vi "Gaussian White Noise (obs 90).vi"(2 "seed":i32=-1, 3 "standard deviation":dbl=1.0000000000000002 format="%0.2f", 4 "samples":i32=128) -> (0 "error":i32, 1 "Gaussian noise pattern":dbl[](array[numeric]))   [LabVIEW 2010, in "NI_AALBase.lvlib"]
doc: "The Gaussian White Noise VI was rewritten in LabVIEW 2009. Replace this VI with a Gaussian White Noise VI from the <B>Functions</B> palette to use the new functionality.\n\nGenerates a Gaussian-distributed, pseudorandom pattern whose statistical profile is (micro,sigma) = (0,s), where s is <B>standard deviation</B>.\n\nThe Gaussian White Noise VI generates the Gaussian-distributed pseudorandom sequence using a modified version of the Box-Muller method to transform uniformly distributed random numbers into Gaussian-distributed random numbers. LabVIEW uses a triple-seeded very-long-cycle linear congruential generation (LCG) algorithm to generate the uniform pseudorandom numbers."
uses:
  NI_AALBase.lvlib
  lvanlys.dll
panel:
  # "Gaussian White Noise"
  # "This VI is obsolete !!!\nYou should replace this VI in your diagram with the Gaussian White Noise VI."
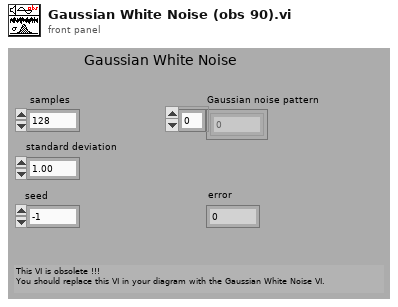
[diagram p1: front panel]
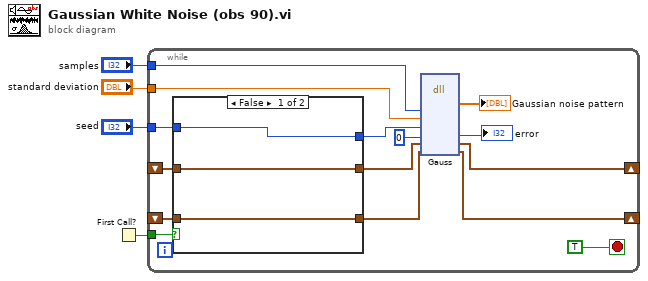
[diagram p0: block diagram]
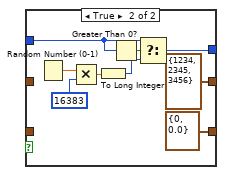
[diagram p2: hidden frame]
diagram:
  n1 = First Call?() -> (First Call?: T/F=w4:bool)
  n2 = while {
    shift-right: [w8] -> _
    shift-left: _ -> [w11]
    tunnel: w4 -> [w5]
    shift-right: [w6] -> _
    shift-left: _ -> [w10]
    tunnel: "seed" -> [w13]
    tunnel: "standard deviation" -> [w15]
    tunnel: "samples" -> [w14]
    stop <- TRUE stop-if-true
    n3 = case shown="False" w5 {
      tunnel: [w21 cluster{"xSeed":i32, "ySeed":i32, "zSeed":i32} {"xSeed"=1234, "ySeed"=2345, "zSeed"=3456} ("RNGState")] -> w9
      tunnel: [w22 w29] -> w12
      tunnel: w13 -> [w22 w30]
      tunnel: [w20 cluster{i32, dbl} {0, 0.0}] -> w7
      tunnel: w11 -> [w21 _]
      tunnel: w10 -> [w20 _]
      frame False {
      }
      frame True {
        n4 = Random Number (0-1)() -> (number: 0 to 1=w27:dbl)
        n5 = Multiply(x=w27, y=16383 ("x")) -> (x*y=w28:dbl)
        n6 = To Long Integer(number=w28) -> (32bit integer=w26:i32)
        n7 = Greater Than 0?(x=w30) -> (x > 0?=w31:bool)
        n8 = Select(t=w30, s=w31, f=w26) -> (s? t:f=w29:i32)
      }
    }
    n9 = dll-call lib="C:/Program Files/National Instruments/LabVIEW 2010/resource/lvanlys.*" fn="Gauss"("size"=w14, "stanDev"=w15, "theSeed"=w12, "dsperr"=0, "rngState"=w9, "gaussState"=w7) -> ("Gaussian noise pattern"=→"Gaussian noise pattern":dbl[], "dsperr"=→"error":i32, "rngState"=w8:cluster{"xSeed":i32, "ySeed":i32, "zSeed":i32}, "gaussState"=w6:cluster{i32, dbl})  [unwired: 4 in, 6 out]
  }
